vi "GetTachometerProperties.vi"(8 "error in (no error)":errorcluster, 11 "Properties":T2[](array[typedef])) -> (0 "error out":errorcluster, 2 "pulses per rev":i32, 3 "Tachometer Config":T1={"slope"=enum."falling", "threshold"=1.0, "hysteresis"=1.0})   [LabVIEW 2017, in "CmsAcquisition.lvlib"]
uses:
  <vilib>/addons/InsightCM/Devices/Shared/Cms/CmsAcquisition/CmsAcquisition.lvlib
  <vilib>/addons/InsightCM/MessageBus/Base/controls/KeyValuePair.ctl
  <vilib>/addons/InsightCM/Devices/Shared/Cms/CmsAcquisition/controls/TachometerConfig.ctl
  <vilib>/addons/InsightCM/Utilities/PropertyHelpers/PropertyHelpers.lvlib
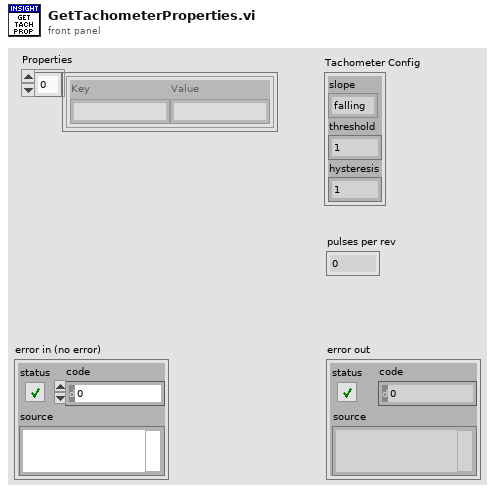
[diagram p1: front panel]
types:
  T1 = typedef "CmsAcquisition.lvlib/TachometerConfig.ctl" = cluster{"slope":enum16{"falling", "rising"}, "threshold":dbl, "hysteresis":dbl}
  T2 = typedef "KeyValuePair.ctl" = cluster{"Key":string, "Value":string}
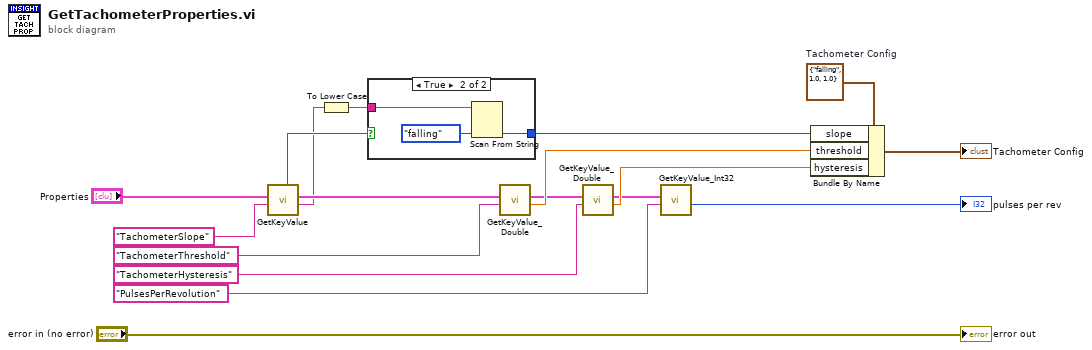
[diagram p0: block diagram]
diagram:
  w18 = T1 {"slope"=enum."falling", "threshold"=1.0, "hysteresis"=1.0}  # Tachometer Config
  n1 = call <vilib>:"GetKeyValue.vi"("key"="TachometerSlope" ("name"), "key value pairs"="Properties") -> ("value"=w8:string, "key value pairs out"=w9:T2[], "found"=w13:bool)  [unwired: 7 in]
  n2 = To Lower Case(string=w8) -> (all lower case string=w17:string)
  n3 = case shown="True" w13 {
    tunnel: w17 -> [_ w20]
    tunnel: [_ w19] -> w16
    frame False {
    }
    frame True {
      n4 = Scan From String(input string=w20, default 1=enum16{"falling", "rising"}."falling" ("slope")) -> (output 1=w19:enum16{"falling", "rising"})  [unwired: 3 in, 3 out]
    }
  }
  n5 = call <vilib>:"GetKeyValue_Double.vi"("key"="TachometerThreshold" ("name"), "key value pairs"=w9) -> ("value"=w12:dbl, "key value pairs out"=w11:T2[])  [unwired: 7 in, 1 out]
  n6 = call <vilib>:"GetKeyValue_Double.vi"("key"="TachometerHysteresis" ("name"), "key value pairs"=w11) -> ("value"=w10:dbl, "key value pairs out"=w3:T2[])  [unwired: 7 in, 1 out]
  n7 = call <vilib>:"GetKeyValue_Int32.vi"("key"="PulsesPerRevolution", "key value pairs"=w3) -> ("value"=→"pulses per rev":i32)  [unwired: 7 in, 2 out]
  n8 = Bundle By Name(cluster=w18, "slope"=w16, "threshold"=w12, "hysteresis"=w10) -> (→"Tachometer Config":T1)
  "error out" <- "error in (no error)"
